vi "Coerce Output Waveforms.vi"(1 "Output Waveforms":waveform(dbl)[](array[waveform])) -> (0 "Coerced Output Waveforms":waveform(dbl)[](array[waveform]))   [LabVIEW 2013]
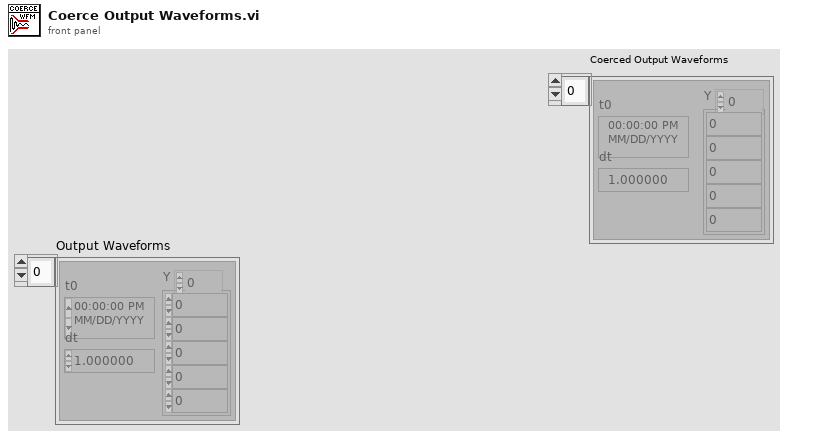
[diagram p1: front panel]
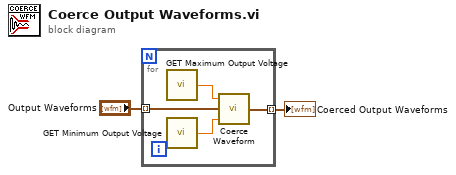
[diagram p0: block diagram]
diagram:
  n1 = for {
    tunnel: "Output Waveforms" -> [w4] mode=indexing
    tunnel: [w3] -> w1 mode=indexing
    n2 = call "GET Maximum Output Voltage.vi"() -> ("Maximum Output Voltage"=w6:dbl)
    n3 = call "GET Minimum Output Voltage.vi"() -> ("Minimum Output Voltage"=w5:dbl)
    n4 = call "Coerce Waveform.vi"("Lower Limit"=w5, "Output Waveform"=w4, "Upper Limit"=w6) -> ("Coerced Output Waveform"=w3:waveform(dbl))
  }
  "Coerced Output Waveforms" <- w1
